vi "Point-in-Quad test.vi"(1 "Point":sgl[](array[numeric]), 2 "Quad":T1) -> (0 "Point is inside quad":bool)   [LabVIEW 2014]
uses:
  Typedefs/Quad.ctl
panel:
  # "PN 17/01/2015"
  # "Vertices"
  # "Edges"
  # "Unit normal"
  # "Edge unit normals"
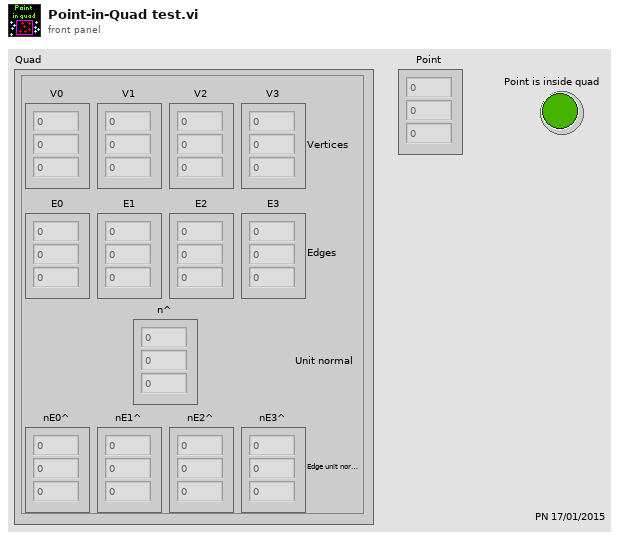
[diagram p1: front panel]
types:
  T1 = typedef "Quad.ctl" = cluster{"V0":sgl[], "V1":sgl[], "V2":sgl[], "V3":sgl[], "E0":sgl[], "E1":sgl[], "E2":sgl[], "E3":sgl[], "n^":sgl[], "nE0^":sgl[], "nE1^":sgl[], "nE2^":sgl[], "nE3^":sgl[]}
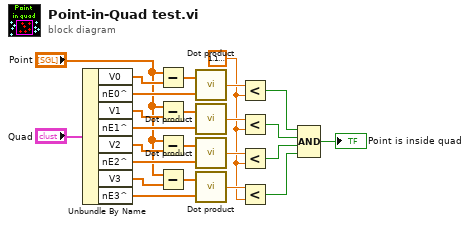
[diagram p0: block diagram]
diagram:
  w6 = sgl 1.1920929e-07
  n1 = Unbundle By Name("Quad") -> ("V0"=w23:sgl[], "nE0^"=w15:sgl[], "V1"=w16:sgl[], "nE1^"=w17:sgl[], "V2"=w19:sgl[], "nE2^"=w18:sgl[], "V3"=w1:sgl[], "nE3^"=w3:sgl[])
  n2 = Subtract(x="Point", y=w23) -> (x-y=w22:sgl[])
  n3 = Subtract(x="Point", y=w16) -> (x-y=w20:sgl[])
  n4 = Subtract(x="Point", y=w19) -> (x-y=w21:sgl[])
  n5 = Subtract(x="Point", y=w1) -> (x-y=w4:sgl[])
  n6 = call "Dot product.vi"("B"=w15, "A"=w22) -> ("A . B"=w14:sgl)
  n7 = call "Dot product.vi"("B"=w17, "A"=w20) -> ("A . B"=w13:sgl)
  n8 = call "Dot product.vi"("B"=w18, "A"=w21) -> ("A . B"=w12:sgl)
  n9 = call "Dot product.vi"("B"=w3, "A"=w4) -> ("A . B"=w7:sgl)
  n10 = Less?(x=w14, y=w6) -> (x < y?=w11:bool)
  n11 = Less?(x=w13, y=w6) -> (x < y?=w10:bool)
  n12 = Less?(x=w12, y=w6) -> (x < y?=w9:bool)
  n13 = Less?(x=w7, y=w6) -> (x < y?=w5:bool)
  n14 = Compound Arithmetic op=AND(w11, w10, w9, w5) -> (→"Point is inside quad":bool)
